vi "Calculate Result Values.vi"(8 "error in":errorcluster, 10 "Signals in":waveform(dbl)[](array[waveform]), 11 "DAC HeatFlow AIV in":refnum<class "DAC HeatFlow AIV.lvclass">) -> (0 "error out":errorcluster, 2 "Signals out":waveform(dbl)[](array[waveform]), 3 "DAC HeatFlow AIV out":refnum<class "DAC HeatFlow AIV.lvclass">)   [LabVIEW 2019, in "DAC.lvlib" / "DAC HeatFlow AIV.lvclass"]
uses:
  DAC HeatFlow AIV.lvclass
  DAC HeatFlow AIV.lvclass/DAC HeatFlow AIV.ctl
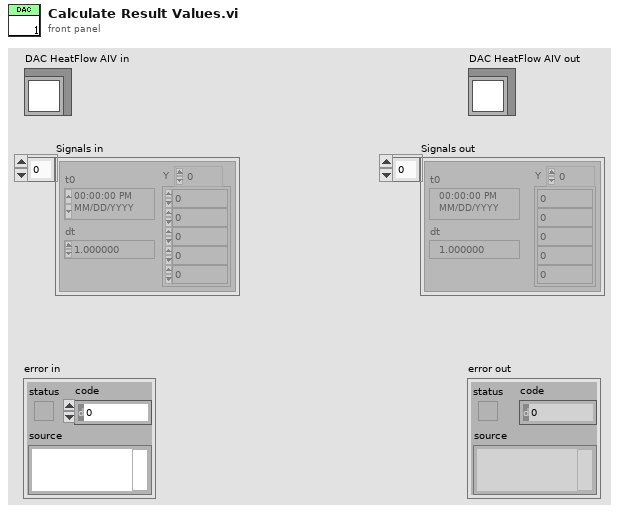
[diagram p1: front panel]
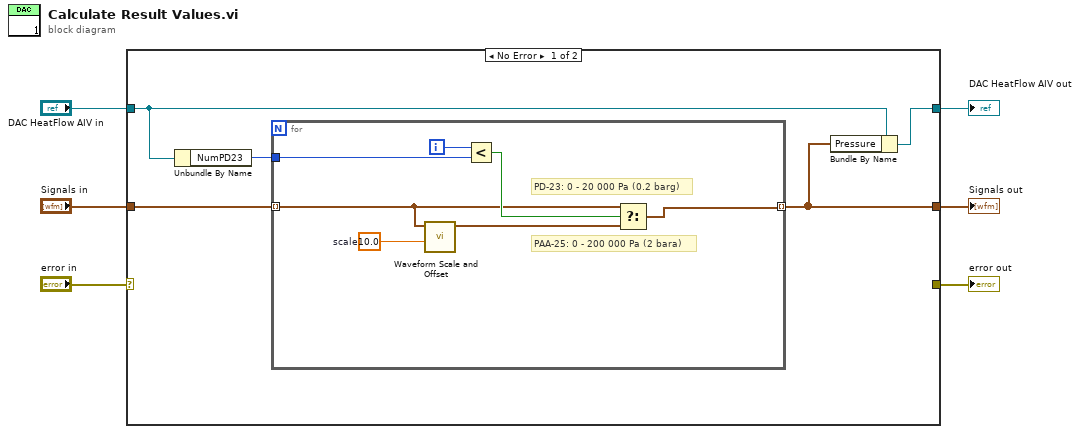
[diagram p0: block diagram]
diagram:
  n1 = case shown="No Error" "error in" {
    selector: "error in" -> [_ w21]
    tunnel: [_ w21] -> w5
    tunnel: [w11 w20] -> w3
    tunnel: "DAC HeatFlow AIV in" -> [w9 w20]
    tunnel: "Signals in" -> [w10 w19]
    tunnel: [w7 w19] -> w1
    frame No Error {
      n2 = Unbundle By Name(w9) -> ("NumPD23"=w8:i32)
      n3 = for {
        tunnel: w10 -> [w15] mode=indexing
        tunnel: w8 -> [w17]
        tunnel: [w12] -> w7 mode=indexing
        i -> [w18]
        w13 = 10.0  # scale
        # "PAA-25: 0 - 200 000 Pa (2 bara)"
        # "PD-23: 0 - 20 000 Pa (0.2 barg)"
        n4 = call <vilib>:"Waveform Scale and Offset.vi"("scale"=w13, "waveform in"=w15) -> ("waveform out"=w14:waveform(dbl))  [unwired: 8 in, 1 out]
        n5 = Less?(x=w18, y=w17) -> (x < y?=w16:bool)
        n6 = Select(t=w15, s=w16, f=w14) -> (s? t:f=w12:waveform(dbl))
      }
      n7 = Bundle By Name(cluster=w9, "Pressure"=w7) -> (w11:refnum<class "DAC HeatFlow AIV.lvclass">)
    }
    frame Error {
    }
  }
  "error out" <- w5
  "DAC HeatFlow AIV out" <- w3
  "Signals out" <- w1
